vi "DoProcess.vi"(8 "error in (no error)":errorcluster, 9 "MsgQ":refnum<queue>, 10 "AbstractionActor.lvclass":refnum<class "AbstractionActor.lvclass">, 11 "ProgramClose in":refnum<class "ProgramClose.lvclass">) -> (0 "error out":errorcluster, 2 "AbstractionActor.lvclass 2":refnum<class "AbstractionActor.lvclass">, 3 "ProgramClose out":refnum<class "ProgramClose.lvclass">)   [LabVIEW 2014, in "ProgramClose.lvclass"]
uses:
  ProgramClose.lvclass
  AbstractionActor/AbstractionActor.lvclass
  AbstractionMessage/AbstractionMessage.lvclass
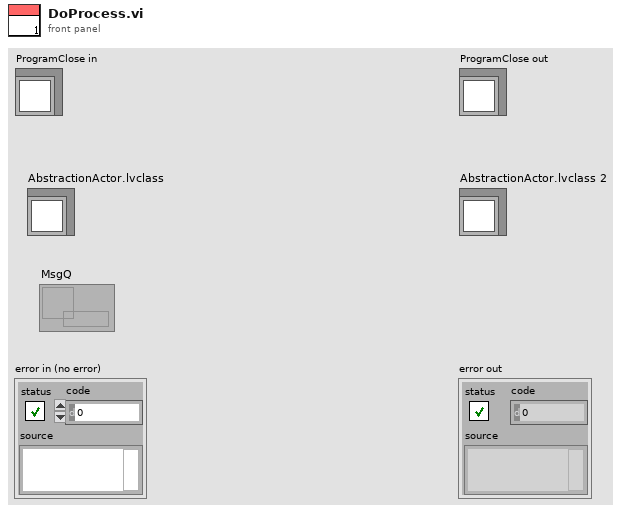
[diagram p1: front panel]
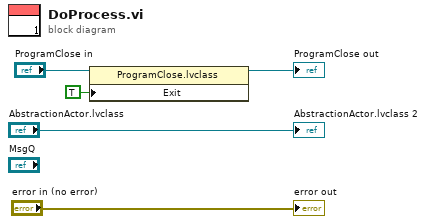
[diagram p0: block diagram]
diagram:
  n1 = property class="ProgramClose.lvclass"(reference="ProgramClose in", "Exit"=TRUE) -> (reference out=→"ProgramClose out":refnum<class "ProgramClose.lvclass">)  [unwired: 1 in, 1 out]
  "error out" <- "error in (no error)"
  "AbstractionActor.lvclass 2" <- "AbstractionActor.lvclass"
